vi "NegateString.vi"(10 "String":string) -> (2 "Negated String":string)   [LabVIEW 2017, in "Transparent Assertions.lvlib" / "LogicalNot.lvclass"]
uses:
  LogicalNot.lvclass
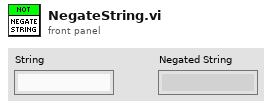
[diagram p1: front panel]
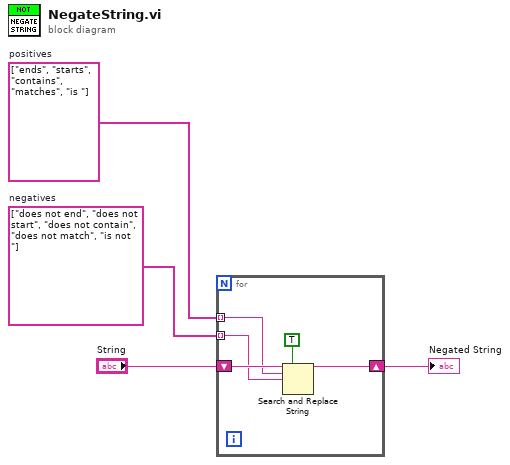
[diagram p0: block diagram]
diagram:
  w1 = string[] ["does not end", "does not start", "does not contain", "does not match", "is not "]  # negatives
  w2 = string[] ["ends", "starts", "contains", "matches", "is "]  # positives
  n1 = for {
    shift-right: [w8] -> w3
    shift-left: "String" -> [w9]
    tunnel: w2 -> [w7] mode=indexing
    tunnel: w1 -> [w6] mode=indexing
    n2 = Search and Replace String(replace all?=TRUE ("replace all? (F)"), input string=w9, search string=w7, replace string=w6) -> (result string=w8:string)  [unwired: 4 in, 3 out]
  }
  "Negated String" <- w3
